vi "9403 Channel Select (SubVI).vi"() -> (0 "error out":errorcluster, 3 "Refnum out":refnum<k21>)   [LabVIEW 2020]
uses:
  <vilib>/DAQmx/create/channels.llb/DAQmx Create Channel (DI-Digital Input).vi
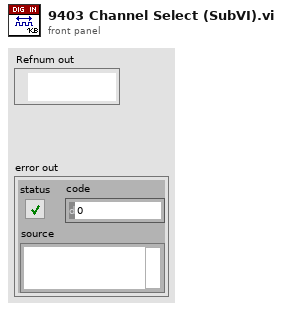
[diagram p1: front panel]
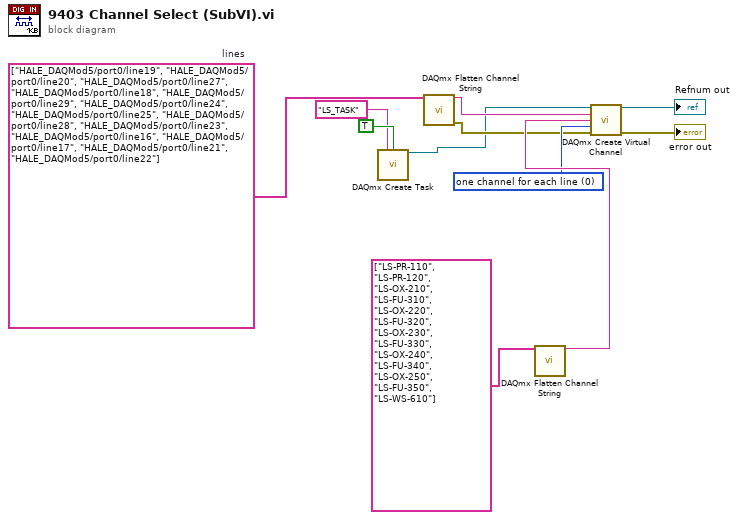
[diagram p0: block diagram]
diagram:
  w4 = tag[] ["HALE_DAQMod5/port0/line19", "HALE_DAQMod5/port0/line20", "HALE_DAQMod5/port0/line27", "HALE_DAQMod5/port0/line18", "HALE_DAQMod5/port0/line29", "HALE_DAQMod5/port0/line24", "HALE_DAQMod5/port0/line25", "HALE_DAQMod5/port0/line28", "HALE_DAQMod5/port0/line23", "HALE_DAQMod5/port0/line16", "HALE_DAQMod5/port0/line17", "HALE_DAQMod5/port0/line21", "HALE_DAQMod5/port0/line22"]  # lines
  w9 = 0 items=["one channel for each line", "one channel for all lines"] ("line grouping")
  n1 = call <vilib>:"DAQmx Create Task.vi"("new task name"="LS_TASK", "auto cleanup"=TRUE) -> ("task out"=w1:refnum<k21>)  [unwired: 12 in, 1 out]
  n2 = call <vilib>:"DAQmx Flatten Channel String.vi"("names in"=w4) -> ("names out"=w5:string, "error out"=w6:errorcluster)  [unwired: 13 in]
  n3 = call <vilib>:"DAQmx Flatten Channel String.vi"("names in"=string[] ["LS-PR-110", "LS-PR-120", "LS-OX-210", "LS-FU-310", "LS-OX-220", "LS-FU-320", "LS-OX-230", "LS-FU-330", "LS-OX-240", "LS-FU-340", "LS-OX-250", "LS-FU-350", "LS-WS-610"] ("name to assign")) -> ("names out"=w11:string)  [unwired: 13 in, 1 out]
  n4 = call-poly <vilib>:"DAQmx Create Virtual Channel.vi"("task in"=w1, "lines"=w5, "name to assign"=w11, "line grouping"=w9, "error in"=w6) -> ("task out"=→"Refnum out":refnum<k21>, "error out"=→"error out":errorcluster)  [unwired: 9 in]
